vi "Teleop.vi"(10 "Match Info":T1={"Autonomous Elapsed Seconds"=0.0, "TeleOp Elapsed Seconds"=0.0, "Disabled Elapsed Seconds"=0.0, "Visited Autonomous"=FALSE, "Visited TeleOp"=FALSE, "Visited Disabled"=FALSE, "Autonomous Settings"={"Autonomous Style"=enum."Independent", "VI Refnum"=refnum}}, 11 "Call Context":T2) -> ()   [LabVIEW 2015]
doc: "This VI is called for each TeleOp packet received from the DS where the robot is not disabled. It is often used to read from the joysticks and update I/O or to update setpoints for timed control loops. It should complete and return within 20 milliseconds or it may miss DS packets."
uses:
  <vilib>/Rock Robotics/WPI/DriverStation/WPI_DriverStationDerivedRobotMode.ctl
  <vilib>/Rock Robotics/WPI/DriverStation/WPI_DriverStationMatch Info.ctl
  <vilib>/Rock Robotics/WPI/Solenoid/WPI_SolenoidValue.ctl
  <vilib>/Rock Robotics/Network Tables/NT Read Boolean.vi
  <vilib>/Rock Robotics/Network Tables/NT Read Number.vi
  <vilib>/Rock Robotics/WPI/Utilities/WPI_GetSetVariantRefNum.vi
  <vilib>/Rock Robotics/WPI/Solenoid/WPI_SolenoidSetEnum.vi
  <vilib>/Rock Robotics/Network Tables/NT Write Boolean.vi
  <vilib>/Rock Robotics/Network Tables/NT Write Number.vi
  <vilib>/addons/control/pid/NI_PID_pid.lvlib
  <vilib>/addons/control/pid/pid.llb/PID (DBL).vi
panel:
  in  "Bras":dbl
  in  "Shifters":dbl
  out "Encodeur gauche min":dbl
  out "Encodeur gauche max":dbl
  out "Encodeur droit max":dbl
  out "Encodeur droit min":dbl
  out "Sample Slider 0":dbl(slide) scale=0.0..5.0
  out "Sample Boolean 1":bool
  out "Sample Boolean 0":bool
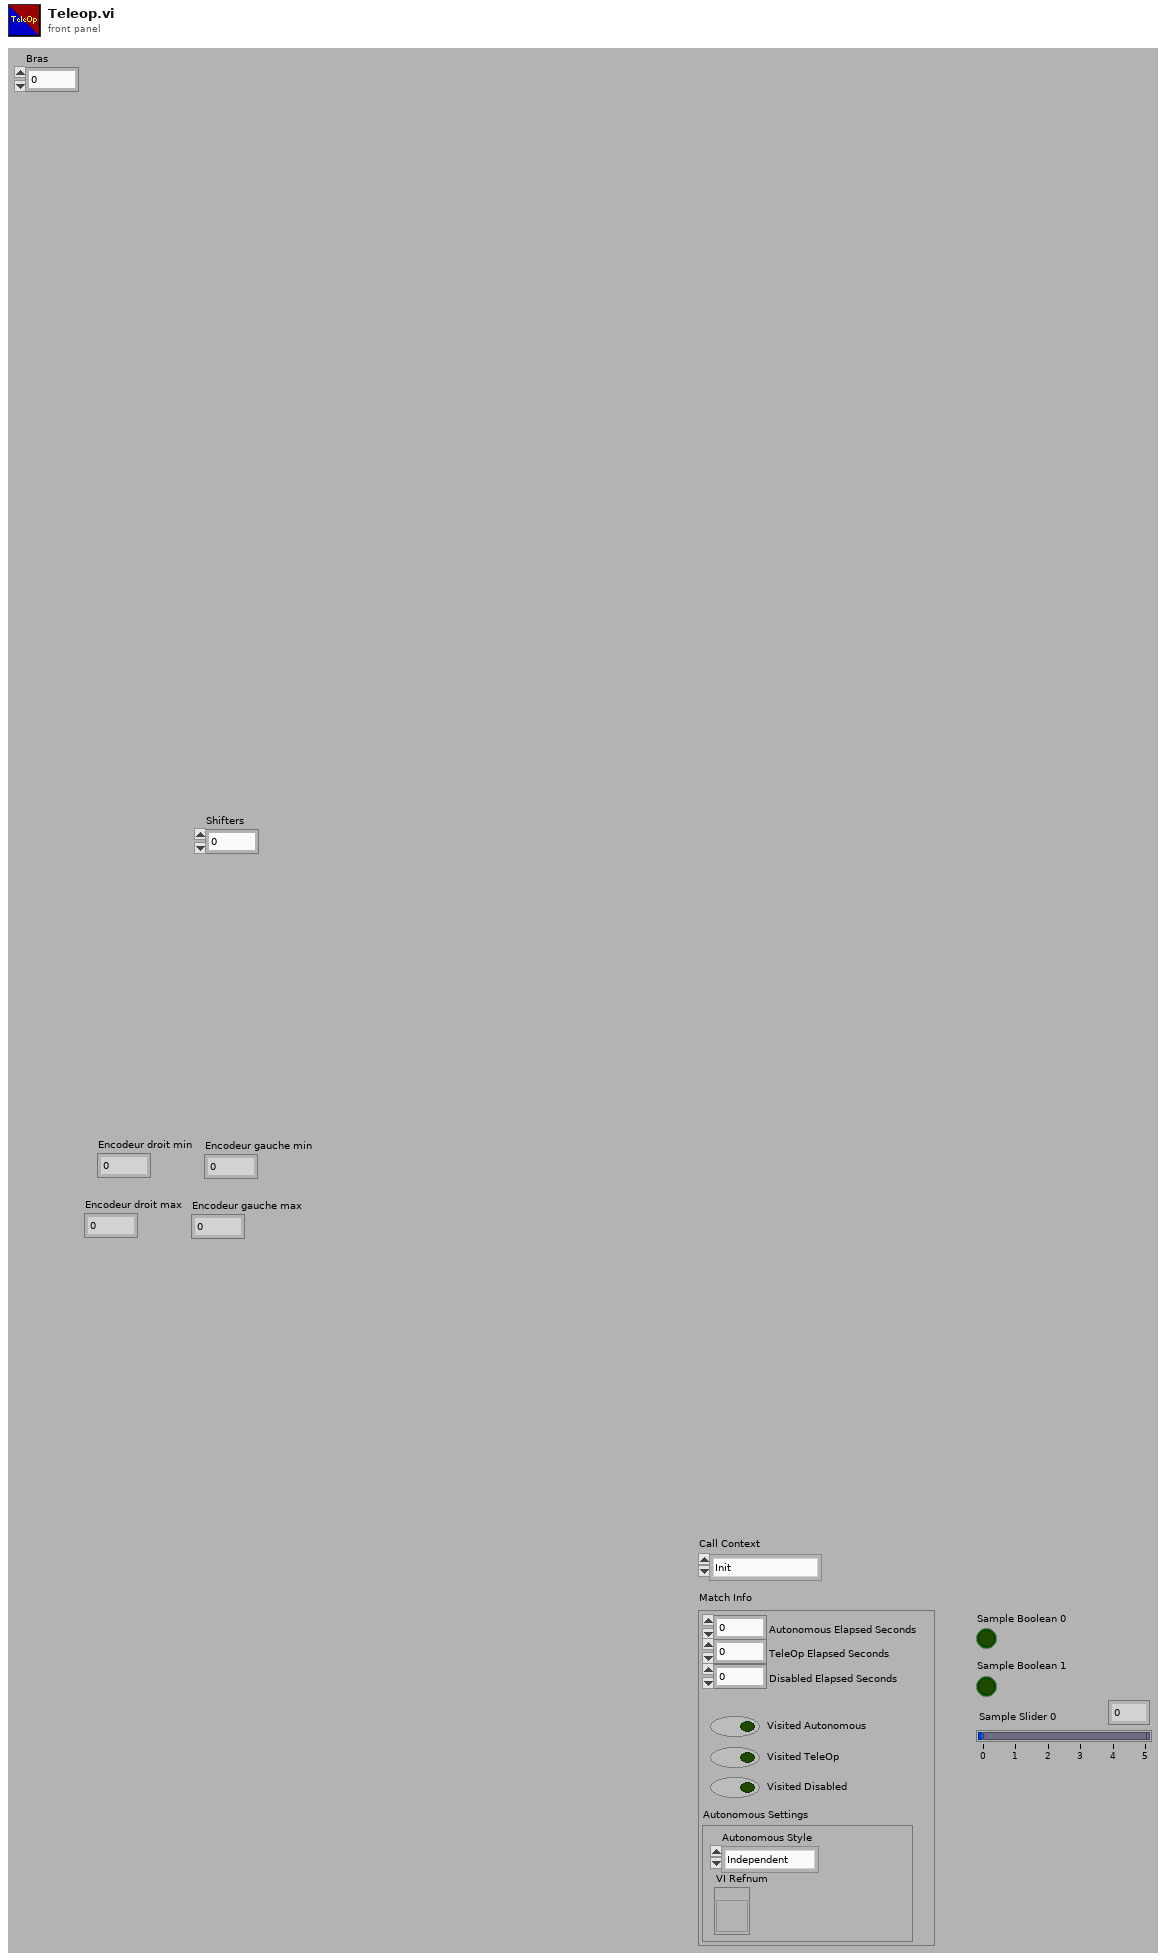
[diagram p1: front panel]
types:
  T1 = typedef "WPI_DriverStationMatch Info.ctl" = cluster{"Autonomous Elapsed Seconds":dbl, "TeleOp Elapsed Seconds":dbl, "Disabled Elapsed Seconds":dbl, "Visited Autonomous":bool, "Visited TeleOp":bool, "Visited Disabled":bool, "Autonomous Settings":cluster{"Autonomous Style":enum16{"Iterative", "Independent"}, "VI Refnum":refnum<vi>}}
  T2 = typedef "WPI_DriverStationDerivedRobotMode.ctl" = enum16{"Init", "Execute", "Stop"}
  T3 = typedef "WPI_JoystickDevRef.ctl" = cluster{"Device":T4}
  T4 = typedef "WPI_JoystickDeviceEnum.ctl" = enum16{"USB 0", "USB 1", "USB 2", "USB 3", "USB 4", "USB 5"}
  T5 = cluster{"Axes[0]":dbl, "Axes[1]":dbl, "Axes[2]":dbl, "Axes[3]":dbl, "Axes[4]":dbl, "Axes[5]":dbl, "Axes[6]":dbl, "Axes[7]":dbl, "Axes[8]":dbl}
  T6 = cluster{"Buttons[0]":bool, "Buttons[1]":bool, "Buttons[2]":bool, "Buttons[3]":bool, "Buttons[4]":bool, "Buttons[5]":bool, "Buttons[6]":bool, "Buttons[7]":bool, "Buttons[8]":bool}
  T7 = typedef "WPI_EncoderDevRef.ctl" = cluster{"DevStatus":errorcluster, "EncoderIndex":T8, "CounterIndex":T9, "DistancePerCount":dbl, "Decoding Type":T10}
  T8 = typedef "FPGA_EncoderIdx.ctl" = enum8{"Enc 0", "Enc 1", "Enc 2", "Enc 3", "Enc 4", "Enc 5", "Enc 6", "Enc 7", "Invalid"}
  T9 = typedef "FPGA_CounterCtrSystemIndex.ctl" = enum8{"Ctr 0", "Ctr 1", "Ctr 2", "Ctr 3", "Ctr 4", "Ctr 5", "Ctr 6", "Ctr 7", "Invalid"}
  T10 = typedef "WPI_EncoderType.ctl" = enum16{"1x", "2x", "4x"}
  T11 = typedef "WPI_SolenoidDevRef.ctl" = cluster{"DevStatus":errorcluster, "Pneumatics Control Module":u8, "Forward Solenoid Channel":T12, "Reverse Solenoid Channel":T12}
  T12 = typedef "WPI_SolenoidChannel.ctl" = enum8{"Solenoid 0", "Solenoid 1", "Solenoid 2", "Solenoid 3", "Solenoid 4", "Solenoid 5", "Solenoid 6", "Solenoid 7", "Invalid"}
  T13 = typedef "WPI_SolenoidValue.ctl" = enum16{"Off", "On", "Forward", "Reverse"}
  T14 = typedef "WPI_MotorControlDeviceRef.ctl" = cluster{"DeviceStatus":errorcluster, "Type":T15, "PWM":cluster{"PWM Channel":T16, "DeadBand":T17}, "CAN":cluster{"Device Number":u8, "Control Mode":T18, "Semaphore":T19, "Max Vout":dbl, "TalonSRX Control Mode":T20}, "Invert":bool}
  T15 = typedef "WPI_MotorControlType.ctl" = enum16{"PWM", "CAN", "CANTalonSRX"}
  T16 = typedef "FPGA_DIOPWMChannel.ctl" = enum8{"PWM 0", "PWM 1", "PWM 2", "PWM 3", "PWM 4", "PWM 5", "PWM 6", "PWM 7", "PWM 8", "PWM 9", "PWM MXP 0", "PWM MXP 1", "PWM MXP 2", "PWM MXP 3", "PWM MXP 4", "PWM MXP 5", "PWM MXP 6", "PWM MXP 7", "PWM MXP 8", "PWM MXP 9", "Invalid"}
  T17 = typedef "WPI_PWMDeadband.ctl" = cluster{"Name":string, "maxPositivePwm":i32, "minPositivePwm":i32, "centerPwm":i32, "maxNegativePwm":i32, "minNegativePwm":i32, "angularRange":u16}
  T18 = typedef "WPI_CANJaguar_ControlMode.ctl" = enum8{"Percent VBus", "Current", "Speed", "Position", "Voltage"}
  T19 = typedef "Semaphore RefNum" = refnum<k1>
  T20 = typedef "WPI_CANTalonSRX_APIControlMode.ctl" = enum8{"Percent VBus", "Speed", "Position", "Slave", "Unchanged / Invalid", "Voltage Compensation", "Current", "Motion Profile"}
  T21 = cluster{"proportional gain (Kc)":dbl, "integral time (Ti, min)":dbl, "derivative time (Td, min)":dbl}
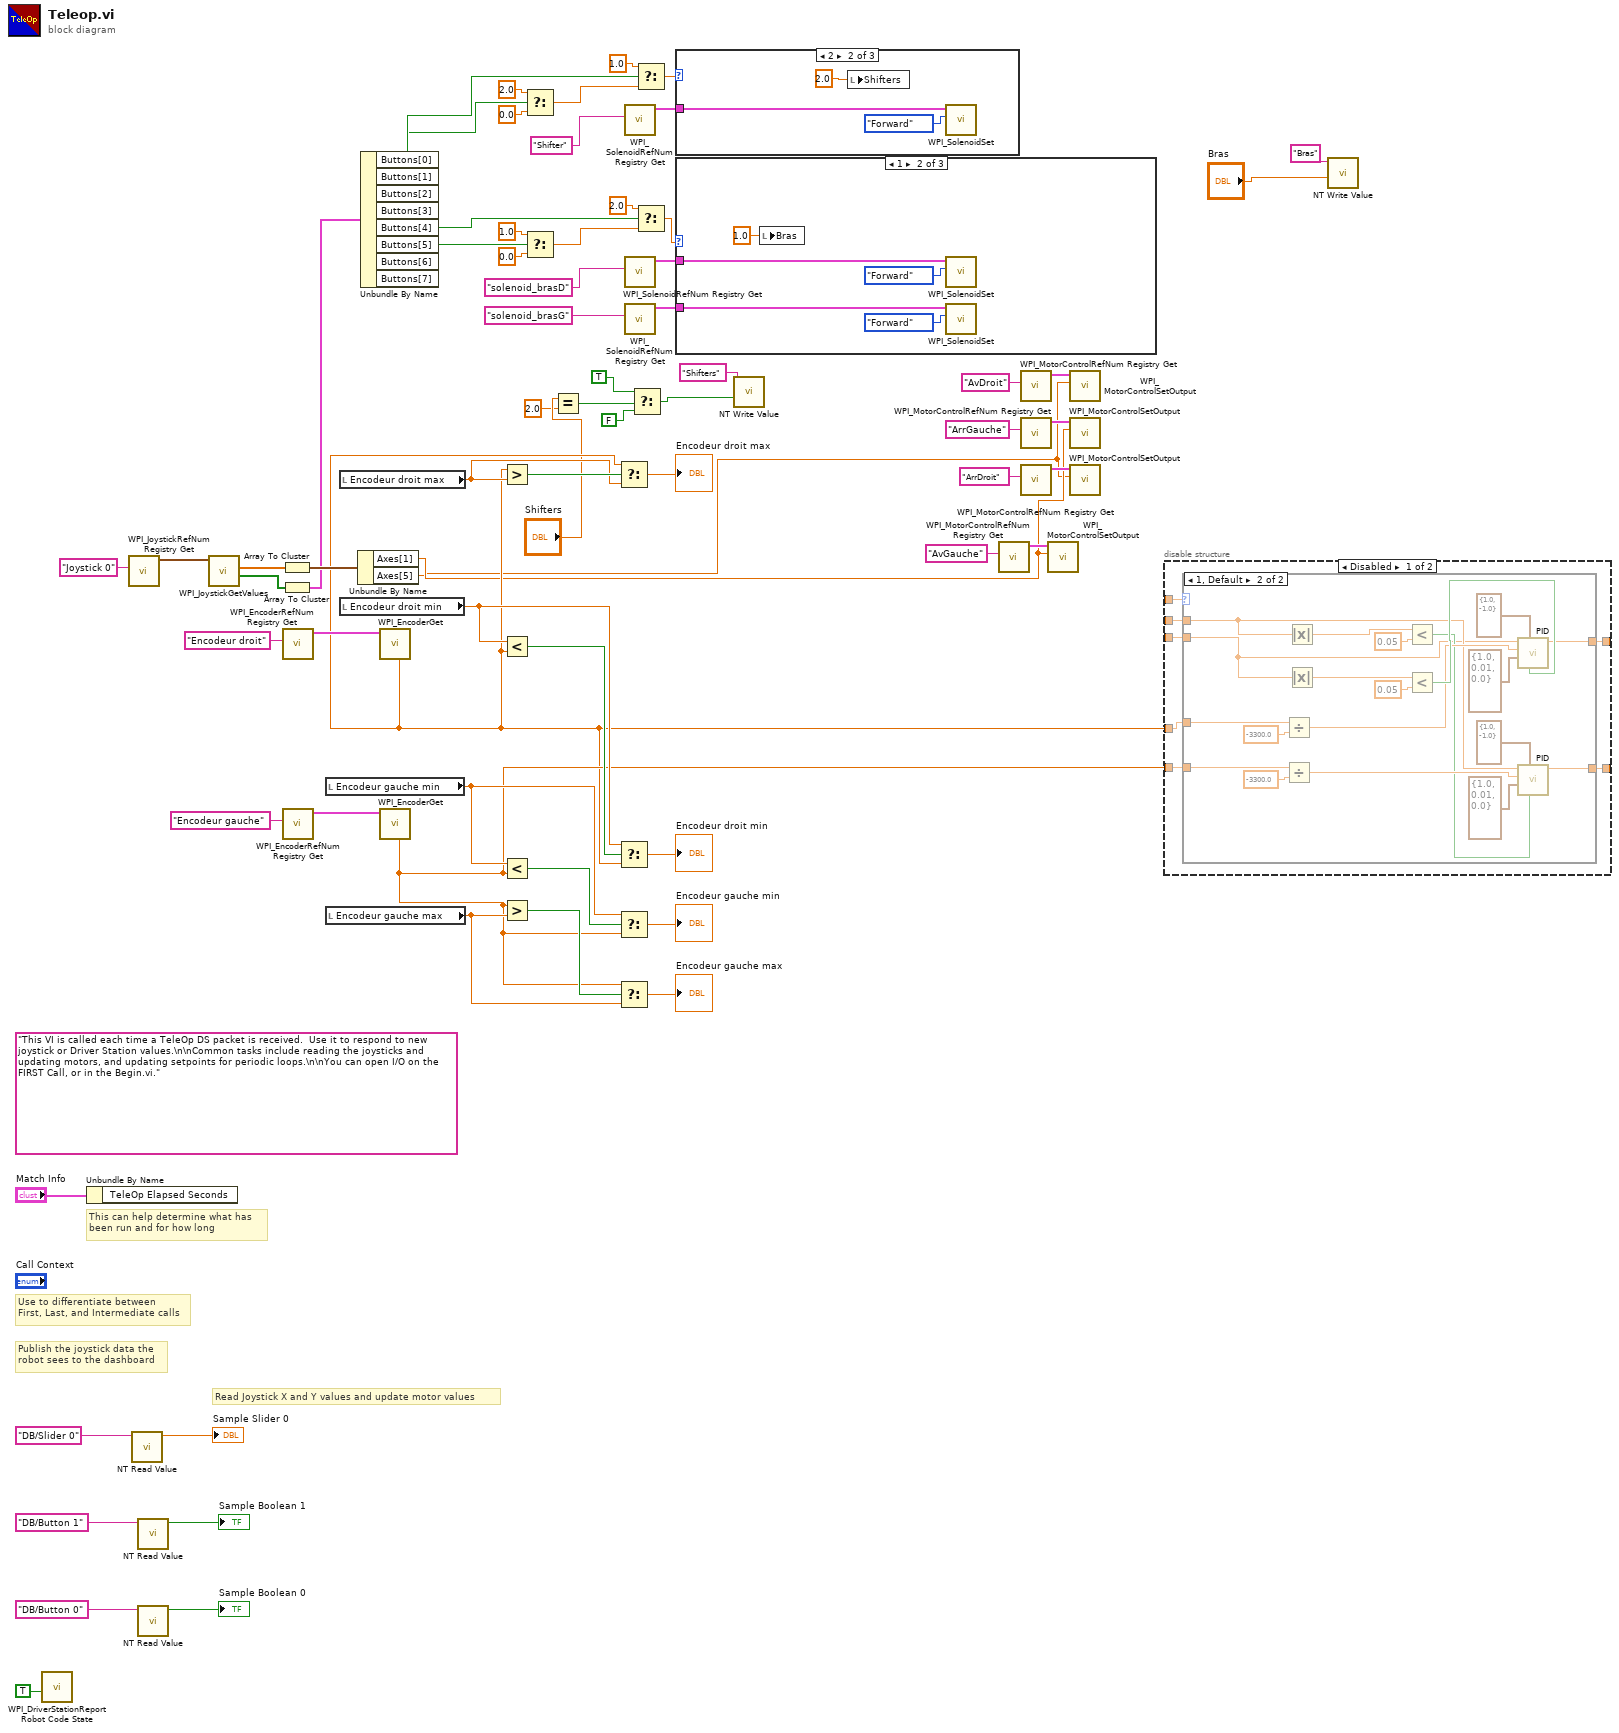
[diagram p0: block diagram]
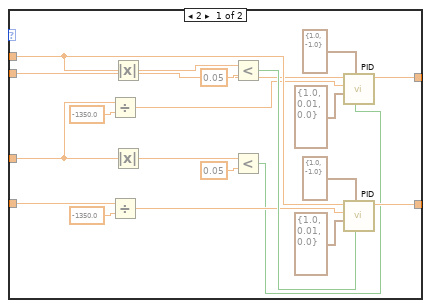
[diagram p2: hidden frame]
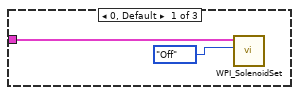
[diagram p4: hidden frame]
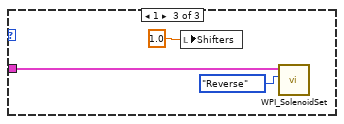
[diagram p5: hidden frame]
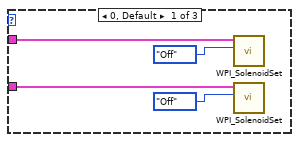
[diagram p6: hidden frame]
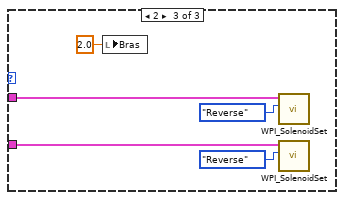
[diagram p7: hidden frame]
diagram:
  (unwired) "This VI is called each time a TeleOp DS packet is received.  Use it to respond to new joystick or Driver Station values.\n\nCommon tasks include reading the joysticks and updating motors, and updating setpoints for periodic loops.\n\nYou can open I/O on the FIRST Call, or in the Begin.vi."
  # "Publish the joystick data the\nrobot sees to the dashboard"
  # "Use to differentiate between\nFirst, Last, and Intermediate calls"
  # "This can help determine what has\nbeen run and for how long"
  # "Read Joystick X and Y values and update motor values"
  n1 = call <vilib>:"WPI_DriverStationReport Robot Code State.vi"("TeleOp"=TRUE ("Autonomous")) -> ()  [unwired: 10 in, 1 out]
  n2 = Unbundle By Name("Match Info") -> ()  [unwired: 1 out]
  n3 = call <vilib>:"WPI_JoystickRefNum Registry Get.vi"("refnum name"="Joystick 0") -> ("JoystickDevRef"=w62:T3)  [unwired: 1 in, 9 out]
  n4 = call-poly <vilib>:"NT Read Value.vi"("Name"="DB/Slider 0" ("refnum name")) -> ("Numeric"=→"Sample Slider 0":dbl)  [unwired: 9 in, 1 out]
  n5 = call-poly <vilib>:"NT Read Value.vi"("Name"="DB/Button 1" ("refnum name")) -> ("Boolean"=→"Sample Boolean 1":bool)  [unwired: 9 in, 1 out]
  n6 = call-poly <vilib>:"NT Read Value.vi"("Name"="DB/Button 0" ("refnum name")) -> ("Boolean"=→"Sample Boolean 0":bool)  [unwired: 9 in, 1 out]
  n7 = call <vilib>:"WPI_JoystickGetValues.vi"("JoystickDevRef"=w62) -> ("Buttons"=w59:bool[], "Axes"=w61:dbl[])  [unwired: 6 in, 3 out]
  n8 = Array To Cluster(array=w61) -> (cluster=w60:T5)
  n9 = Array To Cluster(array=w59) -> (cluster=w16:T6)
  n10 = call <vilib>:"WPI_EncoderRefNum Registry Get.vi"("refnum name"="Encodeur droit") -> ("EncoderDevRef"=w47:T7)  [unwired: 9 in, 1 out]
  n11 = call <vilib>:"WPI_EncoderRefNum Registry Get.vi"("refnum name"="Encodeur gauche") -> ("EncoderDevRef"=w46:T7)  [unwired: 9 in, 1 out]
  n12 = local read "Encodeur gauche min"() -> (w40:dbl)
  n13 = local read "Encodeur gauche max"() -> (w43:dbl)
  n14 = local read "Encodeur droit max"() -> (w38:dbl)
  n15 = local read "Encodeur droit min"() -> (w36:dbl)
  n16 = Unbundle By Name(w60) -> ("Axes[1]"=w2:dbl, "Axes[5]"=w1:dbl)
  n17 = Unbundle By Name(w16) -> ("Buttons[0]"=w15:bool, "Buttons[1]"=w14:bool, "Buttons[4]"=w13:bool, "Buttons[5]"=w12:bool)  [unwired: 4 out]
  n18 = call <vilib>:"WPI_EncoderGet.vi"("EncoderDevRef"=w47) -> ("Rate"=w24:dbl)  [unwired: 5 in, 5 out]
  n19 = call <vilib>:"WPI_EncoderGet.vi"("EncoderDevRef"=w46) -> ("Rate"=w25:dbl)  [unwired: 5 in, 5 out]
  n20 = Greater?(x=w24, y=w38) -> (0:w39:bool)
  n21 = Less?(x=w36, y=w24) -> (x < y?=w37:bool)
  n22 = Less?(x=w40, y=w25) -> (x < y?=w41:bool)
  n23 = Greater?(x=w25, y=w43) -> (0:w44:bool)
  n24 = Select(t=2.0, s=w14, f=0.0) -> (s? t:f=w56:dbl)
  n25 = Select(t=1.0, s=w12, f=0.0) -> (s? t:f=w54:dbl)
  n26 = Equal?(x="Shifters", y=2.0) -> (x = y?=w11:bool)
  n27 = Select(t=w24, s=w39, f=w38) -> (s? t:f=→"Encodeur droit max":dbl)
  n28 = Select(t=w36, s=w37, f=w24) -> (s? t:f=→"Encodeur droit min":dbl)
  n29 = Select(t=w40, s=w41, f=w25) -> (s? t:f=→"Encodeur gauche min":dbl)
  n30 = Select(t=w25, s=w44, f=w43) -> (s? t:f=→"Encodeur gauche max":dbl)
  n31 = call <vilib>:"WPI_SolenoidRefNum Registry Get.vi"("refnum name"="Shifter") -> ("SolenoidDevRef"=w22:T11)  [unwired: 9 in, 1 out]
  n32 = call <vilib>:"WPI_SolenoidRefNum Registry Get.vi"("refnum name"="solenoid_brasD") -> ("SolenoidDevRef"=w17:T11)  [unwired: 9 in, 1 out]
  n33 = call <vilib>:"WPI_SolenoidRefNum Registry Get.vi"("refnum name"="solenoid_brasG") -> ("SolenoidDevRef"=w49:T11)  [unwired: 9 in, 1 out]
  n34 = Select(t=TRUE, s=w11, f=FALSE) -> (s? t:f=w6:bool)
  n35 = Select(t=1.0, s=w15, f=w56) -> (s? t:f=w21:dbl)
  n36 = Select(t=2.0, s=w13, f=w54) -> (s? t:f=w50:dbl)
  n37 = case shown="2" w21 {
    tunnel: w22 -> [w73 w76 w78]
    frame 0, Default {
      n38 = call-poly <vilib>:"WPI_SolenoidSet.vi"("Value"=WPI_SolenoidValue."Off", "SolenoidDevRef"=w73) -> ()  [unwired: 8 in, 2 out]
    }
    frame 2 {
      n39 = local write "Shifters"(2.0 ("Numeric")) -> ()
      n40 = call-poly <vilib>:"WPI_SolenoidSet.vi"("Value"=WPI_SolenoidValue."Forward", "SolenoidDevRef"=w76) -> ()  [unwired: 8 in, 2 out]
    }
    frame 1 {
      n41 = local write "Shifters"(1.0 ("Numeric")) -> ()
      n42 = call-poly <vilib>:"WPI_SolenoidSet.vi"("Value"=WPI_SolenoidValue."Reverse", "SolenoidDevRef"=w78) -> ()  [unwired: 8 in, 2 out]
    }
  }
  n43 = case shown="1" w50 {
    tunnel: w49 -> [w82 w88 w92]
    tunnel: w17 -> [w80 w85 w90]
    frame 0, Default {
      n44 = call-poly <vilib>:"WPI_SolenoidSet.vi"("Value"=WPI_SolenoidValue."Off", "SolenoidDevRef"=w80) -> ()  [unwired: 8 in, 2 out]
      n45 = call-poly <vilib>:"WPI_SolenoidSet.vi"("Value"=WPI_SolenoidValue."Off", "SolenoidDevRef"=w82) -> ()  [unwired: 8 in, 2 out]
    }
    frame 1 {
      n46 = local write "Bras"(1.0 ("Bras")) -> ()
      n47 = call-poly <vilib>:"WPI_SolenoidSet.vi"("Value"=WPI_SolenoidValue."Forward", "SolenoidDevRef"=w85) -> ()  [unwired: 8 in, 2 out]
      n48 = call-poly <vilib>:"WPI_SolenoidSet.vi"("Value"=WPI_SolenoidValue."Forward", "SolenoidDevRef"=w88) -> ()  [unwired: 8 in, 2 out]
    }
    frame 2 {
      n49 = local write "Bras"(2.0 ("Bras")) -> ()
      n50 = call-poly <vilib>:"WPI_SolenoidSet.vi"("Value"=WPI_SolenoidValue."Reverse", "SolenoidDevRef"=w90) -> ()  [unwired: 8 in, 2 out]
      n51 = call-poly <vilib>:"WPI_SolenoidSet.vi"("Value"=WPI_SolenoidValue."Reverse", "SolenoidDevRef"=w92) -> ()  [unwired: 8 in, 2 out]
    }
  }
  n52 = call-poly <vilib>:"NT Write Value.vi"("Boolean"=w6, "Name"="Shifters") -> ()  [unwired: 9 in, 1 out]
  n53 = call <vilib>:"WPI_MotorControlRefNum Registry Get.vi"("refnum name"="AvGauche") -> ("MotorControlDevRef"=w33:T14)  [unwired: 9 in, 1 out]
  n54 = call <vilib>:"WPI_MotorControlRefNum Registry Get.vi"("refnum name"="AvDroit") -> ("MotorControlDevRef"=w31:T14)  [unwired: 9 in, 1 out]
  n55 = call <vilib>:"WPI_MotorControlRefNum Registry Get.vi"("refnum name"="ArrGauche") -> ("MotorControlDevRef"=w32:T14)  [unwired: 9 in, 1 out]
  n56 = call <vilib>:"WPI_MotorControlRefNum Registry Get.vi"("refnum name"="ArrDroit") -> ("MotorControlDevRef"=w30:T14)  [unwired: 9 in, 1 out]
  n57 = call <vilib>:"WPI_MotorControlSetOutput.vi"("Output"=w2, "MotorControlDevRef"=w33) -> ()  [unwired: 7 in, 3 out]
  n58 = call <vilib>:"WPI_MotorControlSetOutput.vi"("Output"=w1, "MotorControlDevRef"=w31) -> ()  [unwired: 7 in, 3 out]
  n59 = call <vilib>:"WPI_MotorControlSetOutput.vi"("Output"=w2, "MotorControlDevRef"=w32) -> ()  [unwired: 7 in, 3 out]
  n60 = call <vilib>:"WPI_MotorControlSetOutput.vi"("Output"=w1, "MotorControlDevRef"=w30) -> ()  [unwired: 7 in, 3 out]
  n61 = disable-structure shown="Disabled" {
    disable-tunnel: w25 -> [w100 _]
    disable-tunnel: w24 -> [w99 _]
    disable-tunnel: _ -> [w98 _]
    disable-tunnel: [w97 _] -> _
    disable-tunnel: _ -> [w96 _]
    disable-tunnel: [w95 _] -> _
    disable-tunnel: _ -> [w94 _]
    frame Disabled {
      n62 = case shown="1, Default" w94 {
        tunnel: w96 -> [w112 w122]
        tunnel: [w113 w126] -> w95
        tunnel: w98 -> [w101 w121]
        tunnel: w99 -> [w102 w123]
        tunnel: [w104 w125] -> w97
        tunnel: w100 -> [w103 w124]
        frame 2 {
          n63 = Divide(x=w102, y=-1350.0) -> (x/y=w107:dbl)
          n64 = Divide(x=w103, y=-1350.0) -> (x/y=w116:dbl)
          n65 = Absolute Value(x=w112) -> (abs(x)=w118:dbl)
          n66 = Absolute Value(x=w102) -> (abs(x)=w109:dbl)
          n67 = Less?(x=w118, y=0.05) -> (x < y?=w120:bool)
          n68 = Less?(x=w109, y=0.05) -> (x < y?=w111:bool)
          n69 = call-poly <vilib>:"PID.vi"("reinitialize? (F)"=w111, "output range"=cluster{"output high":dbl, "output low":dbl} {"output high"=1.0, "output low"=-1.0}, "PID gains"=T21 {"proportional gain (Kc)"=1.0, "integral time (Ti, min)"=0.01, "derivative time (Td, min)"=0.0}, "process variable"=w107, "setpoint"=w101) -> ("output"=w104:dbl)  [unwired: 5 in, 1 out]
          n70 = call-poly <vilib>:"PID.vi"("reinitialize? (F)"=w120, "output range"=cluster{"output high":dbl, "output low":dbl} {"output high"=1.0, "output low"=-1.0}, "PID gains"=T21 {"proportional gain (Kc)"=1.0, "integral time (Ti, min)"=0.01, "derivative time (Td, min)"=0.0}, "process variable"=w116, "setpoint"=w112) -> ("output"=w113:dbl)  [unwired: 5 in, 1 out]
        }
        frame 1, Default {
          n71 = Divide(x=w123, y=-3300.0) -> (x/y=w130:dbl)
          n72 = Divide(x=w124, y=-3300.0) -> (x/y=w137:dbl)
          n73 = Absolute Value(x=w122) -> (abs(x)=w139:dbl)
          n74 = Absolute Value(x=w121) -> (abs(x)=w132:dbl)
          n75 = Less?(x=w139, y=0.05) -> (x < y?=w127:bool)
          n76 = Less?(x=w132, y=0.05) -> (x < y?=w134:bool)
          n77 = call-poly <vilib>:"PID.vi"("reinitialize? (F)"=w134, "output range"=cluster{"output high":dbl, "output low":dbl} {"output high"=1.0, "output low"=-1.0}, "PID gains"=T21 {"proportional gain (Kc)"=1.0, "integral time (Ti, min)"=0.01, "derivative time (Td, min)"=0.0}, "process variable"=w130, "setpoint"=w121) -> ("output"=w125:dbl)  [unwired: 5 in, 1 out]
          n78 = call-poly <vilib>:"PID.vi"("reinitialize? (F)"=w127, "output range"=cluster{"output high":dbl, "output low":dbl} {"output high"=1.0, "output low"=-1.0}, "PID gains"=T21 {"proportional gain (Kc)"=1.0, "integral time (Ti, min)"=0.01, "derivative time (Td, min)"=0.0}, "process variable"=w137, "setpoint"=w122) -> ("output"=w126:dbl)  [unwired: 5 in, 1 out]
        }
      }
    }
    frame Enabled {
    }
  }
  n79 = call-poly <vilib>:"NT Write Value.vi"("Numeric"="Bras", "Name"="Bras") -> ()  [unwired: 9 in, 1 out]
